vi "Termometr.vi"() -> ()   [LabVIEW 2023]
uses:
  <vilib>/numeric/Random Number (Range) U64.vi
  <vilib>/numeric/sub_Random U32.vi
panel:
  in  "stop":bool
  in  "Skala":bool
  out "Temperatura [F]":dbl(slide) scale=0.0..100.0
  out "Temperatura [C]":dbl(slide) scale=0.0..30.0
  # "Deg C"
  # "Deg F"
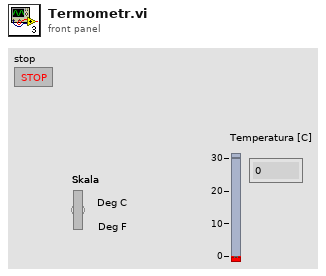
[diagram p1: front panel]
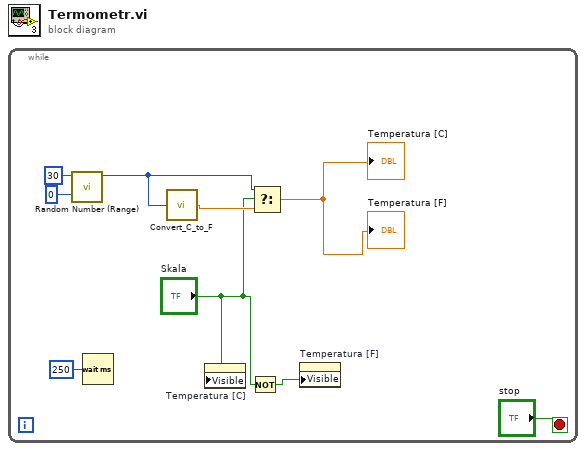
[diagram p0: block diagram]
diagram:
  n1 = while {
    stop <- "stop" stop-if-true
    n2 = call-poly <vilib>:"Random Number (Range).vi"("lower bound (0)"=u64 0, "upper bound (100)"=u64 30) -> ("number"=w6:u64)  [unwired: 9 in]
    n3 = Wait (ms)(milliseconds to wait=u32 250) -> ()  [unwired: 1 out]
    n4 = call "Convert_C_to_F.vi"("deg C"=w6) -> ("deg F"=w7:dbl)
    n5 = property on="Temperatura [C]" class="Slide (strict)"("Visible"="Skala") -> ()  [unwired: 2 in, 2 out]
    n6 = Not(x="Skala") -> (.not. x?=w4:bool)
    n7 = Select(t=w6, s="Skala", f=w7) -> (s? t:f=→"Temperatura [C]" →"Temperatura [F]":dbl)
    n8 = property on="Temperatura [F]" class="Slide (strict)"("Visible"=w4) -> ()  [unwired: 2 in, 2 out]
  }
